vi "initialise.vi"(8 "error in (no error)":errorcluster, 11 "SignalReaderDL091205FPGA in":refnum<class "SignalReaderDL091205FPGA.lvclass">) -> (0 "error out":errorcluster, 3 "SignalReaderDL091205FPGA out":refnum<class "SignalReaderDL091205FPGA.lvclass">)   [LabVIEW 2010, in "SignalReaderDL091205FPGA.lvclass"]
doc: "The dynamic dispatch-version of this VI initalises the plug-in object by allocating and initalising any dynamic resources need."
uses:
  SignalReaderDL091205FPGA.lvclass
  GenericSignalReader/GenericSignalReader/GenericSignalReader.lvclass
  SignalReaderDL091205FPGA.lvclass/SignalReaderDL091205FPGA.ctl
  FPGAWrapper/GenericFPGAWrapper/GenericFPGAWrapper/GenericFPGAWrapper.lvclass
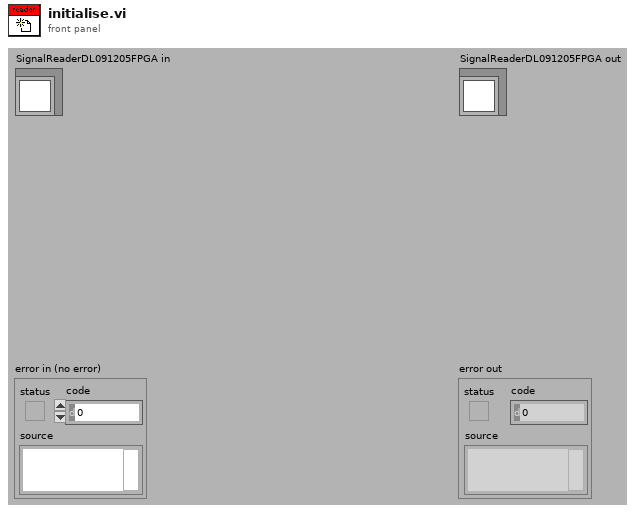
[diagram p1: front panel]
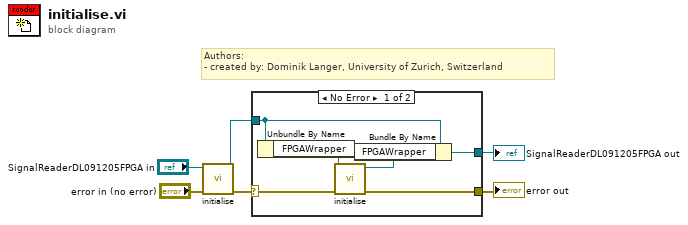
[diagram p0: block diagram]
diagram:
  # "Authors: \n- created by: Dominik Langer, University of Zurich, Switzerland"
  n1 = call-parent "initialise.vi"("error in (no error)"="error in (no error)", "GenericPlugin in"="SignalReaderDL091205FPGA in") -> ("error out"=w4:errorcluster, "GenericPlugin out"=w3:refnum<class "SignalReaderDL091205FPGA.lvclass">)  [unwired: 8 in]
  n2 = case shown="No Error" w4 {
    selector: w4 -> [w12 w13]
    tunnel: w3 -> [w10 w14]
    tunnel: [w8 w13] -> w1
    tunnel: [w7 w14] -> w2
    frame No Error {
      n3 = Unbundle By Name(w10) -> ("FPGAWrapper"=w11:refnum<class "GenericFPGAWrapper.lvclass">)
      n4 = call-dynamic "initialise.vi"("error in (no error)"=w12, "GenericPlugin in"=w11) -> ("error out"=w8:errorcluster, "GenericPlugin out"=w9:refnum<class "GenericFPGAWrapper.lvclass">)  [unwired: 8 in]
      n5 = Bundle By Name(cluster=w10, "FPGAWrapper"=w9) -> (w7:refnum<class "SignalReaderDL091205FPGA.lvclass">)
    }
    frame Error {
    }
  }
  "error out" <- w1
  "SignalReaderDL091205FPGA out" <- w2
